vi "CLOSE CONNECTION.vi"(8 "error in (no error)":errorcluster) -> (0 "error out":errorcluster)   [LabVIEW 2025]
uses:
  CAMERA CODE/POST ANALYSIS ENUM.ctl
  CAMERA CODE/CAMERA LIVE FEED ENUM.ctl
  9f89fbd5-d746-4d8c-8908-f8483b521604.vi
  789754c0-7336-4ae4-af50-f9468950345a.vi
  29cf5344-e428-46d5-8dbd-f9476090f9e6.vi
  7eaf8574-cd07-49d6-83de-007bc696c653.vi
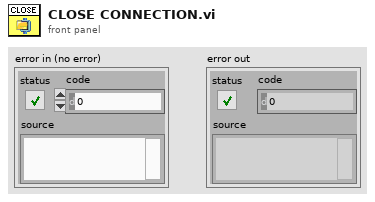
[diagram p1: front panel]
types:
  T1 = typedef "POST ANALYSIS ENUM.ctl" = enum16{"OPEN EXE", "INIT", "OPEN FILE", "FIT", "DRAW REC", "DRAW LINE", "PAN", "ZOOM IN", "ZOOM OUT", "SET ZOOM", "CLEAR ROI", "GET MEASUREMENTS", "RESIZE MODE", "STREAM START", "STREAM STOP", "SHOW UI", "MINIMIZE UI", "HIDE UI", "CKISE APP", "CLOSE CONNECTION", "SAVE IMAGE", "SET ROI COLOR", "READ", "TCP CHECK", "CLOSE"}
  T2 = typedef "CAMERA LIVE FEED ENUM.ctl" = enum16{"OPEN EXE", "INIT", "READ", "CAMERA CONNECT", "CAMERA START", "CAMERA STOP", "CAMERA GRAY", "CAMERA RGB", "CAMERA MINIMIZE", "CAMERA CLOSE", "CAMERA MODE LIST", "CAMERA MODE SET", "CAMERA RESTORE", "CAMERA SAVE", "CLOSE"}
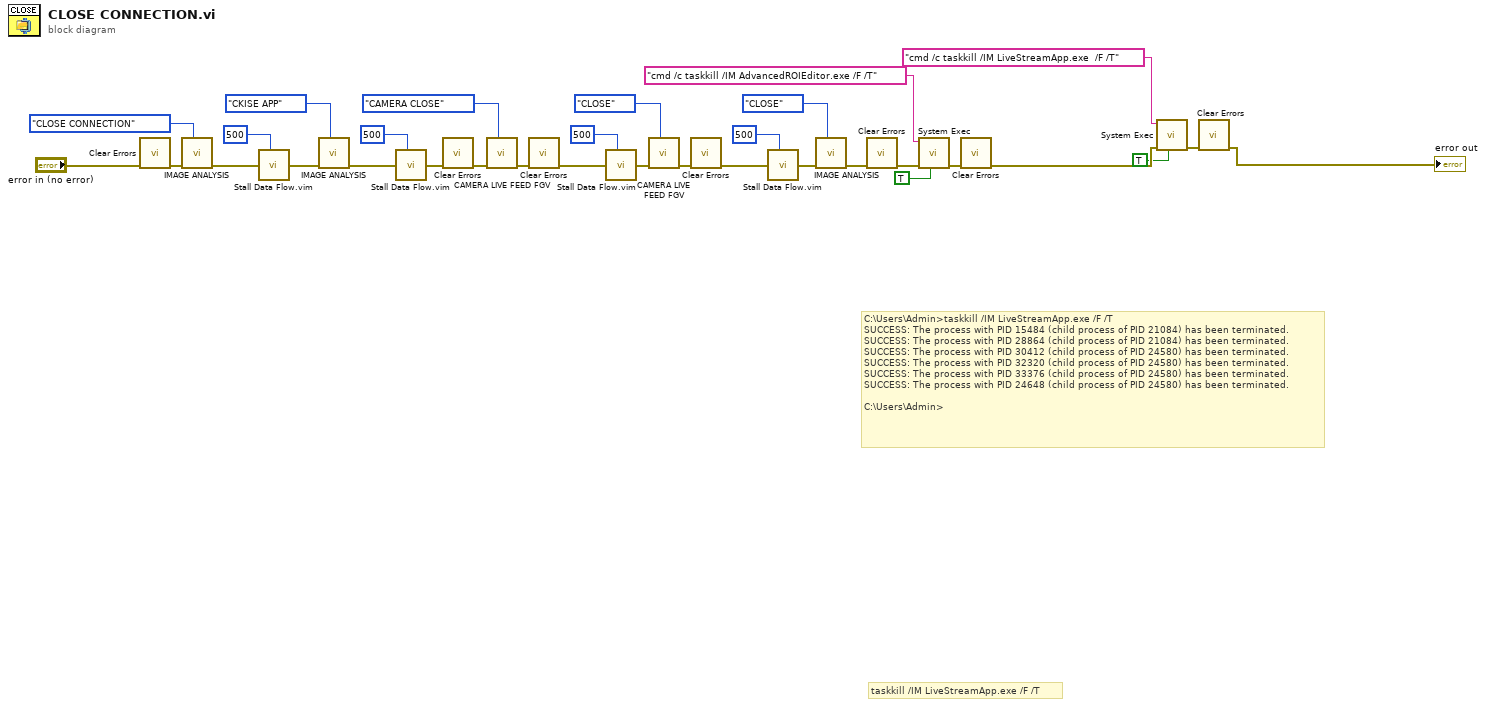
[diagram p0: block diagram]
diagram:
  # "taskkill /IM LiveStreamApp.exe /F /T"
  # "C:\\Users\\Admin>taskkill /IM LiveStreamApp.exe /F /T\nSUCCESS: The process with PID 15484 (child process of PID 21084) has been terminated.\nSUCCESS: The process with PID 28864 (child process of PID 21084) has been terminated.\nSUCCESS: The process with PID 30412 (child process of PID 24580) has been terminated.\nSUCCESS: The process with PID 32320 (child process of PID 24580) has been terminated.\nSUCCESS: The process with PID 33376 (child process of PID 24580) has been terminated.\nSUCCESS: The process with PID 24648 (child process of PID 24580) has been terminated.\n\nC:\\Users\\Admin>"
  n1 = call <vilib>:"Clear Errors.vi"("error in (no error)"="error in (no error)") -> ("error out"=w28:errorcluster)  [unwired: 5 in, 1 out]
  n2 = call "IMAGE ANALYSIS.vi"("Enum"=POST_ANALYSIS_ENUM."CLOSE CONNECTION", "error in"=w28) -> ("error out"=w25:errorcluster)  [unwired: 8 in, 1 out]
  n3 = call "Stall Data Flow.vim"("value in"=w25, "milliseconds to wait"=u32 500) -> ("value out"=w23:errorcluster)  [unwired: 1 out]
  n4 = call "IMAGE ANALYSIS.vi"("Enum"=POST_ANALYSIS_ENUM."CKISE APP", "error in"=w23) -> ("error out"=w21:errorcluster)  [unwired: 8 in, 1 out]
  n5 = call "Stall Data Flow.vim"("value in"=w21, "milliseconds to wait"=u32 500) -> ("value out"=w20:errorcluster)  [unwired: 1 out]
  n6 = call <vilib>:"Clear Errors.vi"("error in (no error)"=w20) -> ("error out"=w30:errorcluster)  [unwired: 5 in, 1 out]
  n7 = call "CAMERA LIVE FEED FGV.vi"("Enum - Menu"=CAMERA_LIVE_FEED_ENUM."CAMERA CLOSE", "error in (no error)"=w30) -> ("error out"=w29:errorcluster)  [unwired: 8 in, 1 out]
  n8 = call <vilib>:"Clear Errors.vi"("error in (no error)"=w29) -> ("error out"=w16:errorcluster)  [unwired: 5 in, 1 out]
  n9 = call "Stall Data Flow.vim"("value in"=w16, "milliseconds to wait"=u32 500) -> ("value out"=w18:errorcluster)  [unwired: 1 out]
  n10 = call "CAMERA LIVE FEED FGV.vi"("Enum - Menu"=CAMERA_LIVE_FEED_ENUM."CLOSE", "error in (no error)"=w18) -> ("error out"=w14:errorcluster)  [unwired: 8 in, 1 out]
  n11 = call <vilib>:"Clear Errors.vi"("error in (no error)"=w14) -> ("error out"=w10:errorcluster)  [unwired: 5 in, 1 out]
  n12 = call "Stall Data Flow.vim"("value in"=w10, "milliseconds to wait"=u32 500) -> ("value out"=w13:errorcluster)  [unwired: 1 out]
  n13 = call "IMAGE ANALYSIS.vi"("Enum"=POST_ANALYSIS_ENUM."CLOSE", "error in"=w13) -> ("error out"=w11:errorcluster)  [unwired: 8 in, 1 out]
  n14 = call <vilib>:"Clear Errors.vi"("error in (no error)"=w11) -> ("error out"=w9:errorcluster)  [unwired: 5 in, 1 out]
  n15 = call <vilib>:"System Exec.vi"("run minimized? (F)"=TRUE, "error in (no error)"=w9, "command line"="cmd /c taskkill /IM AdvancedROIEditor.exe /F /T") -> ("error out"=w8:errorcluster)  [unwired: 5 in, 3 out]
  n16 = call <vilib>:"Clear Errors.vi"("error in (no error)"=w8) -> ("error out"=w4:errorcluster)  [unwired: 5 in, 1 out]
  n17 = call <vilib>:"System Exec.vi"("run minimized? (F)"=TRUE, "error in (no error)"=w4, "command line"="cmd /c taskkill /IM LiveStreamApp.exe  /F /T") -> ("error out"=w5:errorcluster)  [unwired: 5 in, 3 out]
  n18 = call <vilib>:"Clear Errors.vi"("error in (no error)"=w5) -> ("error out"=→"error out":errorcluster)  [unwired: 5 in, 1 out]
